vi "TRITON_GET_STATUS.vi"(3 "error in (no error)":errorcluster, 5 "Response String":string) -> (0 "error out":errorcluster, 2 "Status":string)   [LabVIEW 2019]
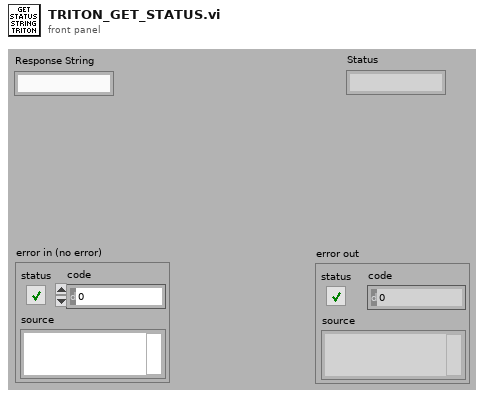
[diagram p1: front panel]
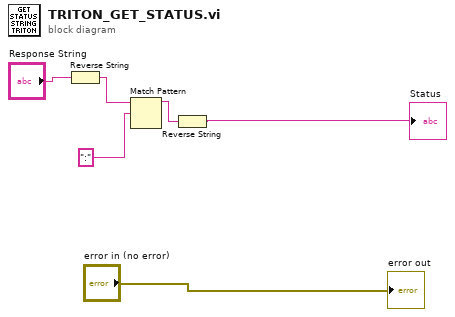
[diagram p0: block diagram]
diagram:
  n1 = Reverse String(1:"Response String") -> (0:w6:string)
  n2 = Match Pattern(string=w6, regular expression=":") -> (before substring=w4:string)  [unwired: 1 in, 3 out]
  n3 = Reverse String(1:w4) -> (0:→"Status":string)
  "error out" <- "error in (no error)"
